vi "Variant attributes experiment.vi"() -> ()   [LabVIEW 2011]
uses:
  <vilib>/Utility/GetType.llb/Type Enum.ctl
  JSON Value/JSON Value.lvclass
  Variant JSON/Variant JSON.lvlib
panel:
  out "Type Enum":T1=enum."String"
  out "String":string
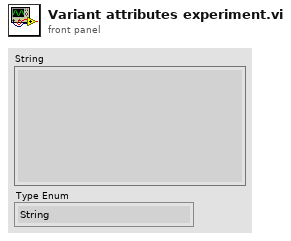
[diagram p1: front panel]
types:
  T1 = typedef "Type Enum.ctl" = enum8{"Void", "I8", "I16", "I32", "I64", "U8", "U16", "U32", "U64", "Single Float", "Double Float", "Extended Float", "Single Complex", "Double Complex", "Extended Complex", "Enum I8 NEVER", "Enum I16 NEVER", "Enum I32 NEVER", "Enum I64 NEVER", "Enum U8", "Enum U16", "Enum U32", "Enum U64", "Single Float With Unit", "Double Float With Unit", "Extended Float With Unit", "Single Complex With Unit", "Double Complex With Unit", "Extended Complex With Unit", "boolU16", "Boolean", "String", "Handle", "Path", "Picture", "C String", "Pascal String", "Tag", "SubString", "Array", "SubArray", "Cluster", "Numeric Cluster", "Variant", "LV Variant", "Measure Data (waveform)", "Refnum", "ExtData", "function", "Typedef", "Poly VI", "bad wire", "LabVIEW Class Instance"}
  T2 = cluster{"VariantAttributes":variant, "EmptyVariant":variant}
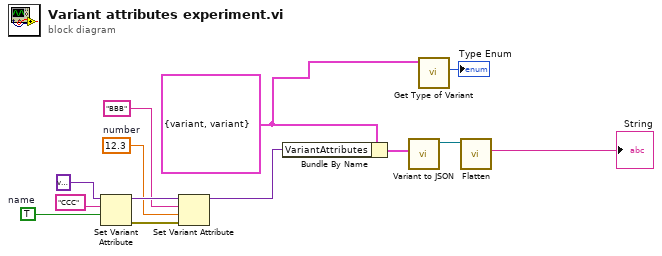
[diagram p0: block diagram]
diagram:
  w5 = 12.3  # number
  w2 = T2 {"VariantAttributes"=variant, "EmptyVariant"=variant}
  w11 = TRUE  # name
  n1 = Set Variant Attribute(Variant=variant ("variant"), name="CCC", value=w11) -> (Variant out=w7:variant, error out=w8:errorcluster)  [unwired: 1 in, 1 out]
  n2 = Set Variant Attribute(Variant=w7, name="BBB", value=w5, error in=w8) -> (Variant out=w6:variant)  [unwired: 2 out]
  n3 = Bundle By Name(cluster=w2, "VariantAttributes"=w6) -> (w9:T2)
  n4 = call "Variant to JSON.vi"("Variant"=w9) -> ("JSON Value out"=w13:refnum<class "JSON Value.lvclass">)  [unwired: 9 in, 1 out]
  n5 = call <vilib>:"Get Type of Variant.vi"("Data In"=w2) -> ("Type Enum"=→"Type Enum":T1)  [unwired: 9 in, 1 out]
  n6 = call-dynamic "Flatten.vi"("JSON Value in"=w13) -> ("String"=→"String":string)  [unwired: 9 in, 1 out]
